vi "DLL Path FG.vi"(10 "Set? (F)":bool, 11 "DLL Path In":path) -> (3 "DLL Path":path)   [LabVIEW 2022 SP3, in "VoiceMeeterRemote.lvlib"]
uses:
  VoiceMeeterRemote.lvlib
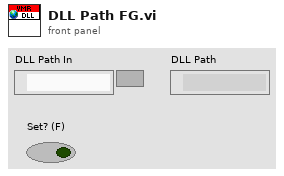
[diagram p1: front panel]
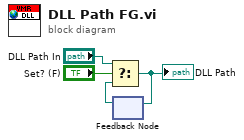
[diagram p0: block diagram]
diagram:
  n1 = feedback #1() -> (w2:path)  [unwired: 1 in]
  n2 = Select(t="DLL Path In", s="Set? (F)", f=w2) -> (s? t:f=w1:path)
  "DLL Path" <- w1
  n3 = feedback-in #1(w1) -> ()
